vi "RT Loop - Analyze Acceleration_11.vi"(7 "testing":bool, 8 "error in (no error)":errorcluster, 9 "Acceleration RT FIFO In":T1, 10 "FPGA VI Reference Out 2":refnum<k20>, 11 "Message Queue":refnum<queue>) -> (1 "Acceleration RT FIFO Out":T1)   [LabVIEW 2017]
doc: "Read and analyze acceleration waveform data from FPGA via DMA FIFO. If the acceleration is over the limit, then send the acceleration waveform data to the Log Data Loop."
uses:
  UI Error Handlers/support/Message Queue/Message Cluster.ctl
  controls/Acceleration RT FIFO Reference.ctl
  Globals/Global - All RT Loop Stop.vi
  Globals/Global - Configuration Options.vi
  <vilib>/Utility/error.llb/Error Cluster From Error Code.vi
  <vilib>/rvi/errors/niLvFpgaAdjustHostInterfaceError.vi
  <vilib>/rvi/interface/nirviMethod/nirviMethod.xnode
  <vilib>/FPGAPlugInAG/Dynamic/niLvFpga_ReadFifo_Dynamic.vi
  <vilib>/rvi/errors/niLvFpgaMergeErrorWithErrorCode.vi
  UI Error Handlers/support/Message Queue/Message Queue.lvlib
panel:
  out "x-y":u32
  out "G1 status.G1 trigger":bool
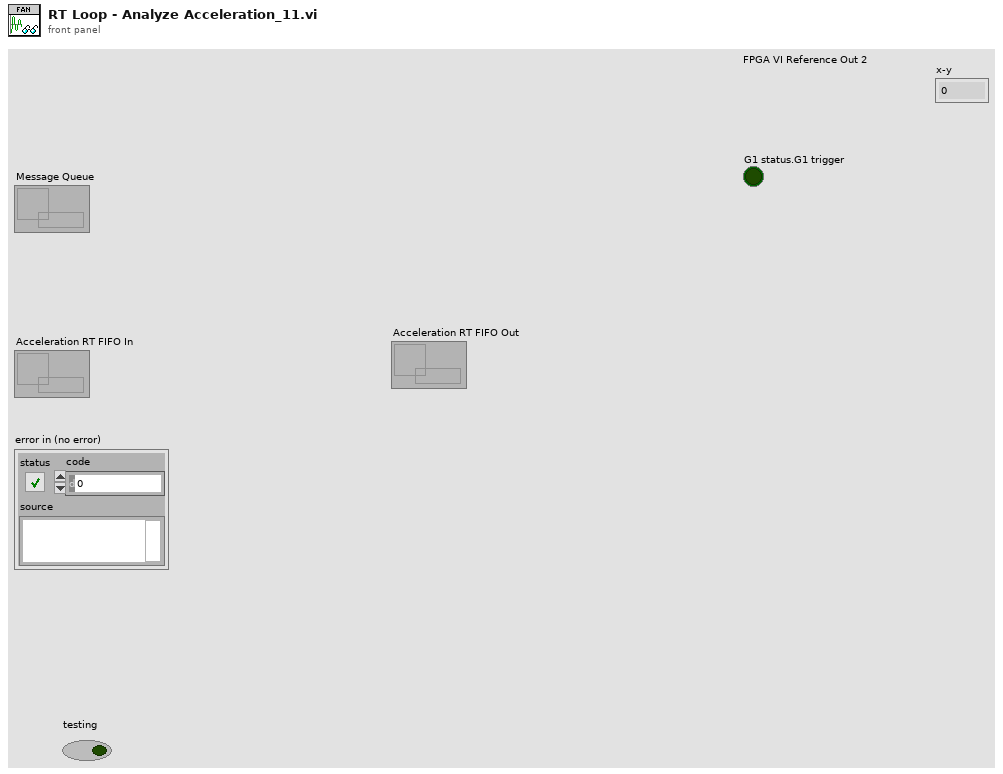
[diagram p1: front panel]
types:
  T1 = typedef "Acceleration RT FIFO Reference.ctl" = refnum<k33>
  T2 = cluster{"Tool data":cluster{"Number of teeth":sgl}, "Cutting data":cluster{"rpm":sgl}, "Limits":cluster{"Magnitude threshold":sgl, "Tolerance":sgl}, "G1 status":cluster{"G1 trigger":bool}}
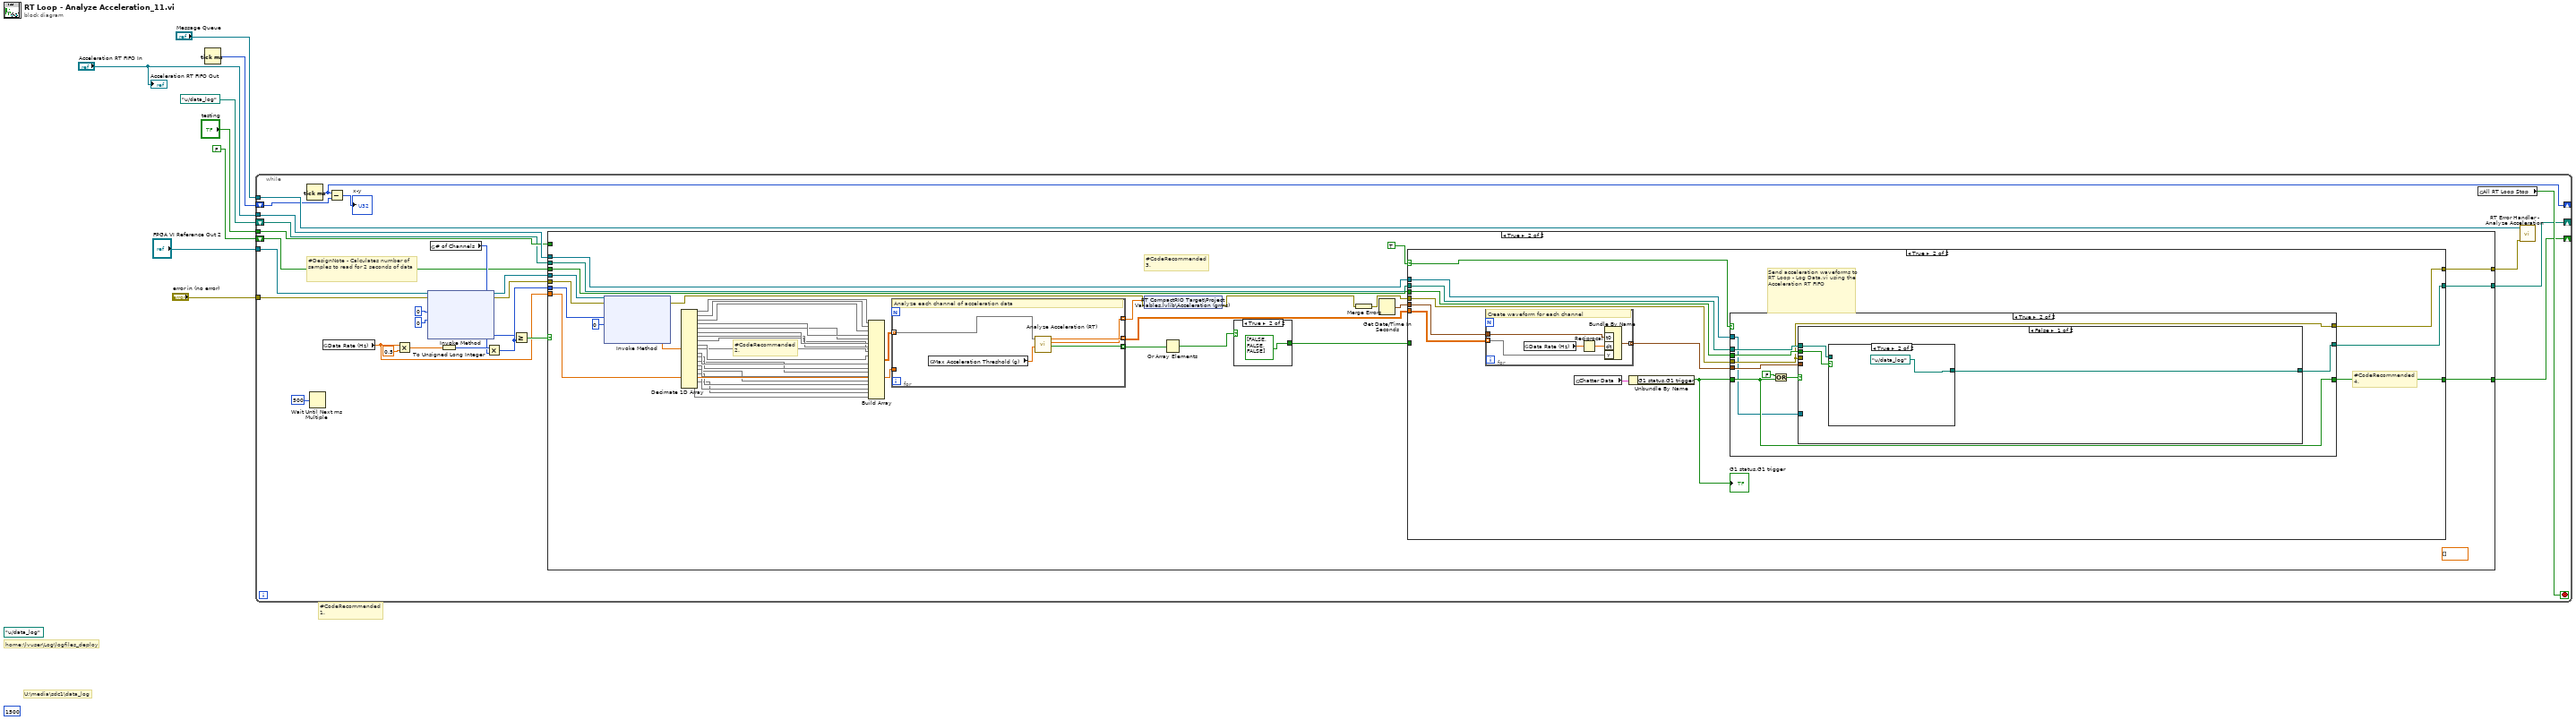
[diagram p0: block diagram]
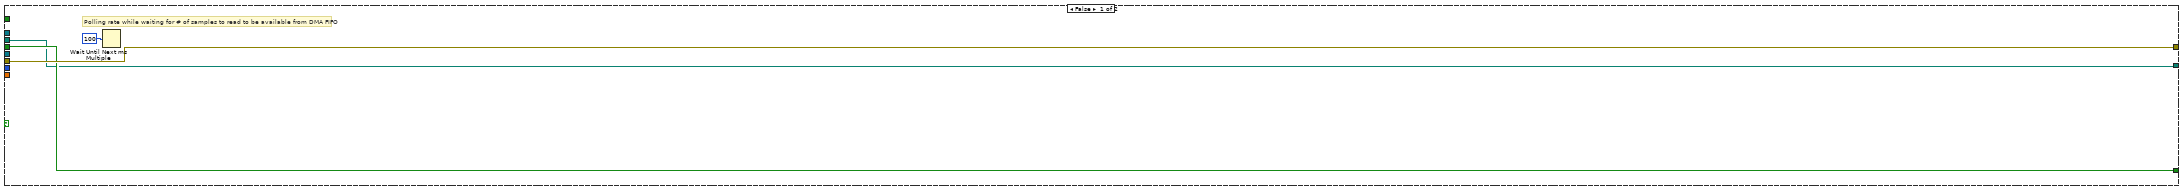
[diagram p2: hidden frame]
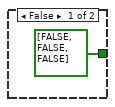
[diagram p3: hidden frame]
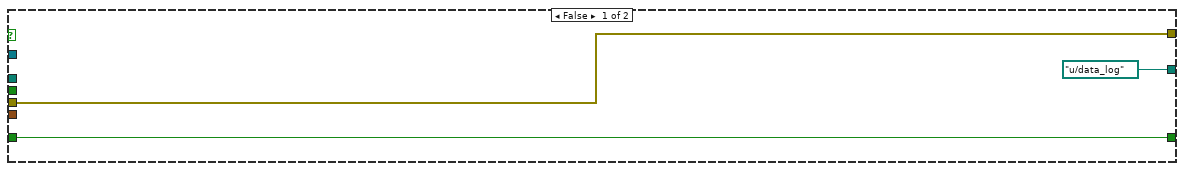
[diagram p5: hidden frame]
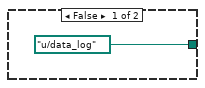
[diagram p6: hidden frame]
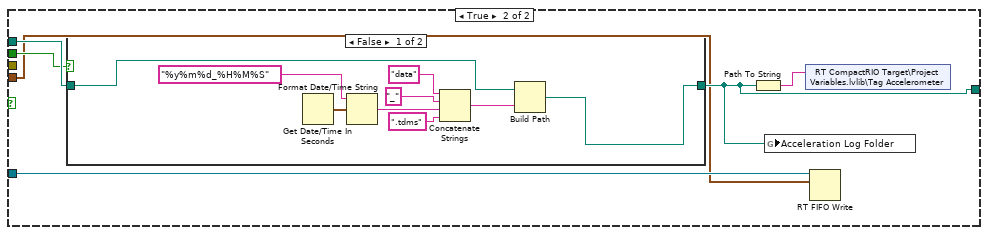
[diagram p7: hidden frame]
diagram:
  (unwired) 1500 ("max queue size (-1, unlimited)")
  (unwired) path "u:/data_log" ("AVI Path")
  # "U:\\media\\sdc1\\data_log"
  # "home:\\lvuser\\Log\\logfiles_deploy"
  # "#CodeRecommended\n1."
  n1 = Tick Count (ms)() -> (millisecond timer value=w2:u32)
  n2 = while {
    tunnel: "FPGA VI Reference Out 2" -> [w35]
    tunnel: "error in (no error)" -> [w34]
    tunnel: "Message Queue" -> [w27]
    tunnel: "Acceleration RT FIFO In" -> [w25]
    tunnel: "testing" -> [w17]
    shift-right: [w14] -> _
    shift-left: path "u:/data_log" ("AVI Path") -> [w13]
    shift-right: [w16] -> _
    shift-left: FALSE -> [w15]
    shift-right: [w11] -> _
    shift-left: w2 -> [w12]
    stop <- w28 stop-if-true
    # "#DesignNote - Calculates number of samples to read for 2 seconds of data"
    n3 = Tick Count (ms)() -> (millisecond timer value=w11:u32)
    n4 = Wait Until Next ms Multiple(millisecond multiple=u32 500) -> ()  [unwired: 1 out]
    n5 = global read "Global - Configuration Options.vi" "Data Rate (Hz)"() -> (w19:dbl)
    n6 = Subtract(x=w11, y=w12) -> (x-y=→"x-y":u32)
    n7 = Multiply(x=w19, y=0.5) -> (x*y=w23:dbl)
    n8 = xnode "Invoke Method"("FPGA VI Reference In"=w35, "error in"=w34, "Number of Elements"=u32 0, "Timeout (ms)"=0) -> ("FPGA VI Reference Out"=w31:refnum<k20>, "error out"=w30:errorcluster, "Elements Remaining"=w18:u32)  [unwired: 1 out]
    n9 = global read "Global - Configuration Options.vi" "# of Channels"() -> (w20:u32)
    n10 = To Unsigned Long Integer(number=w23) -> (unsigned 32bit integer=w22:u32)
    n11 = Multiply(x=w22, y=w20) -> (x*y=w21:u32)
    n12 = Greater Or Equal?(x=w18, y=w21) -> (x >= y?=w29:bool)
    n13 = case shown="True" w29 {
      tunnel: w31 -> [_ w81]
      tunnel: w30 -> [w39 w80]
      tunnel: [w39 w76] -> w26
      tunnel: w21 -> [_ w79]
      tunnel: w25 -> [_ w74]
      tunnel: w19 -> [_ w71]
      tunnel: w17 -> [_ _]
      tunnel: [w37 w65] -> w16
      tunnel: w15 -> [w37 w64]
      tunnel: [w36 w63] -> w14
      tunnel: w13 -> [w36 w62]
      frame False {
        # "Polling rate while waiting for # of samples to read to be available from DMA FIFO"
        n14 = Wait Until Next ms Multiple(millisecond multiple=u32 100) -> ()  [unwired: 1 out]
      }
      frame True {
        (unwired) dbl[] []
        # "#CodeRecommended\n3."
        # "#CodeRecommended\n2."
        n15 = xnode "Invoke Method"("FPGA VI Reference In"=w81, "error in"=w80, "Number of Elements"=w79, "Timeout (ms)"=0) -> ("error out"=w70:errorcluster, "Data"=w73:sgl[])  [unwired: 2 out]
        n16 = Decimate 1D Array(w73) -> (w59:sgl[], w58:sgl[], w57:sgl[], w55:sgl[], w54:sgl[], w53:sgl[], w52:sgl[], w51:sgl[], w50:sgl[], w49:sgl[], w48:sgl[], w47:sgl[], w46:sgl[], w45:sgl[], w44:sgl[], w43:sgl[], w42:sgl[], w41:sgl[], w40:sgl[])
        n17 = Build Array(w59, w58, w57, w55, w54, w53, w52, w51, w50, w49, w48, w47, w46, w45, w44, w43, w42, w41, w40) -> (w60:sgl[][])
        n18 = for {
          tunnel: [w88] -> w75 mode=indexing
          tunnel: [w87] -> w72 mode=indexing
          tunnel: [w86] -> w56 mode=indexing
          tunnel: w71 -> [_]
          tunnel: w60 -> [w84] mode=indexing
          # "Analyze each channel of acceleration data"
          n19 = global read "Global - Configuration Options.vi" "Max Acceleration Threshold (g)"() -> (w85:sgl)
          n20 = call "Analyze Acceleration (RT).vi"("Max Instantaneous Acceleration (g)"=w85, "Acceleration Waveform (SGL)"=w84) -> ("Over Limit?"=w88:bool, "Acceleration (grms)"=w86:dbl, "Acceleration Waveform (DBL)"=w87:dbl[])  [unwired: 7 in]
        }
        n21 = shared-variable "RT CompactRIO Target\\Project Variables.lvlib\\Acceleration (grms)"(w56, error in=w70) -> (error out=w69:errorcluster)
        n22 = Or Array Elements(Boolean array=w75) -> (logical OR=w67:bool)
        n23 = case shown="True" w67 {
          tunnel: [bool[] [FALSE, FALSE, FALSE] ("Chatter?") bool[] [FALSE, FALSE, FALSE] ("Chatter?")] -> w66
          frame False {
          }
          frame True {
          }
        }
        n24 = Merge Errors(w69) -> (w68:errorcluster)
        n25 = Get Date/Time In Seconds() -> (seconds since 1Jan1904=w77:timestamp)
        n26 = case shown="True" TRUE {
          selector: TRUE -> [_ w92]
          tunnel: w77 -> [_ w104]
          tunnel: w68 -> [w91 w103]
          tunnel: [w91 w93] -> w76
          tunnel: w74 -> [_ w101]
          tunnel: w72 -> [_ w100]
          tunnel: w66 -> [_ _]
          tunnel: [w90 w98] -> w65
          tunnel: w64 -> [w90 w97]
          tunnel: [w89 w96] -> w63
          tunnel: w62 -> [w89 w94]
          frame False {
          }
          frame True {
            # "#CodeRecommended\n4."
            # "Send acceleration waveforms to RT Loop - Log Data.vi using the Acceleration RT FIFO"
            n27 = for {
              tunnel: w100 -> [w142] mode=indexing
              tunnel: w104 -> [w141]
              tunnel: [w139] -> w102 mode=indexing
              # "Create waveform for each channel"
              n28 = global read "Global - Configuration Options.vi" "Data Rate (Hz)"() -> (w138:dbl)
              n29 = Reciprocal(x=w138) -> (1/x=w140:dbl)
              n30 = Bundle By Name("t0"=w141, "dt"=w140, "Y"=w142) -> (w139:waveform(dbl))  [unwired: 1 in]
            }
            n31 = global read "Global - Configuration Options.vi" "Chatter Data"() -> (w99:T2)
            n32 = Unbundle By Name(w99) -> ("G1 status.G1 trigger"=w95:bool)
            "G1 status.G1 trigger" <- w95
            n33 = case shown="True" w92 {
              tunnel: w103 -> [w107 w109]
              tunnel: w102 -> [_ w110]
              tunnel: w101 -> [_ w108]
              tunnel: w95 -> [w106 w114]
              tunnel: [w106 w114] -> w98
              tunnel: w97 -> [_ w113]
              tunnel: [path "u:/data_log" ("AVI Path") w112] -> w96
              tunnel: w94 -> [_ w111]
              tunnel: [w107 w109] -> w93
              frame False {
              }
              frame True {
                n34 = Or(x=FALSE, y=w114) -> (x .or. y?=w116:bool)
                n35 = case shown="False" w116 {
                  tunnel: w111 -> [w117 w127]
                  tunnel: [w119 w124] -> w112
                  tunnel: w113 -> [w118 w126]
                  tunnel: w110 -> [_ w122]
                  tunnel: w109 -> [_ _]
                  tunnel: w108 -> [_ w123]
                  frame False {
                    n36 = case shown="True" w118 {
                      tunnel: [path "u:/data_log" ("AVI Path") path "u:/data_log" ("AVI Path")] -> w119
                      tunnel: w117 -> [_ _]
                      frame False {
                      }
                      frame True {
                      }
                    }
                  }
                  frame True {
                    n37 = case shown="False" w126 {
                      tunnel: w127 -> [w129 w137]
                      tunnel: [w128 w137] -> w124
                      frame False {
                        n38 = Get Date/Time In Seconds() -> (seconds since 1Jan1904=w132:timestamp)
                        n39 = Format Date/Time String(time format string (%c)="%y%m%d_%H%M%S", seconds (now)=w132) -> (date/time string=w135:string)  [unwired: 1 out]
                        n40 = Concatenate Strings("data" ("string"), "_" ("string"), w135, ".tdms" ("string")) -> (w130:string)
                        n41 = Build Path(base path=w129, name or relative path=w130) -> (appended path=w128:path)
                      }
                      frame True {
                      }
                    }
                    n42 = Path To String(path=w124) -> (string=w125:string)
                    n43 = global write "Global - Configuration Options.vi" "Acceleration Log Folder"(w124) -> ()
                    n44 = shared-variable "RT CompactRIO Target\\Project Variables.lvlib\\Tag Accelerometer"(w125) -> ()  [unwired: 1 in, 1 out]
                    n45 = RT FIFO Write(0:w123, 1:w122) -> ()  [unwired: 3 in, 4 out]
                  }
                }
              }
            }
          }
        }
      }
    }
    n46 = global read "Global - All RT Loop Stop.vi" "All RT Loop Stop"() -> (w28:bool)
    n47 = call "RT Error Handler - Analyze Acceleration.vi"("error in (no error)"=w26, "Message Queue"=w27) -> ()  [unwired: 9 in, 1 out]
  }
  "Acceleration RT FIFO Out" <- "Acceleration RT FIFO In"
